vi "LXY_step.vi"() -> ()   [LabVIEW 2019]
uses:
  lib/Keithley 622x/Configure/2182 -A/Low Level/Typedefs/KE2182 -- Voltage Ranges.ctl
  lib/Keithley 622x/Configure/2182 -A/Low Level/Typedefs/KE2182 -- Filter Type.ctl
  lib/Keithley 622x/Configure/2182 -A/Low Level/Typedefs/KE2182 -- Filter Count.ctl
  lib/Keithley 622x/Configure/2182 -A/Low Level/Typedefs/KE2182 -- Filter Window.ctl
  lib/Keithley 622x/Configure/2182 -A/Low Level/Typedefs/KE2182 -- NPLCs.ctl
  lib/Keithley 622x/Configure/Delta PDelta DCon Modes/Typedefs/KE622x -- Delta Mode Params.ctl
  lib/Keithley 622x/Configure/Delta PDelta DCon Modes/Low Level/Typedefs/KE622x -- Delta PDelta Mode High Level.ctl
  lib/Keithley 622x/Configure/Delta PDelta DCon Modes/Low Level/Typedefs/KE622x -- Delta PDelta Mode Low Level.ctl
  lib/Keithley 622x/Configure/Delta PDelta DCon Modes/Low Level/Typedefs/KE622x -- Delta DCon Mode Delay.ctl
  lib/Keithley 622x/Configure/Delta PDelta DCon Modes/Low Level/Typedefs/KE622x -- Delta PDelta Mode Num Cycles Mode.ctl
  lib/Keithley 622x/Configure/Delta PDelta DCon Modes/Low Level/Typedefs/KE622x -- Delta PDelta Mode Num Cycles.ctl
  SubVI/ctl/config.ctl
  <vilib>/NI/Modbus Library/API/Master/Modbus Master.lvclass
  SubVI/ctl/initialize.ctl
  SubVI/ctl/Instrument.ctl
  SubVI/ctl/Instrument Type.ctl
  D:/measure/lib/QDInstrument.dll
  lib/QDInstrument.dll
  SubVI/ctl/335 state.ctl
  SubVI/ctl/limit.ctl
  SubVI/ctl/9T mag field stauts.ctl
  SubVI/ctl/warning.ctl
  lib/Keithley 622x/Keithley 622x.lvlib
panel:
  in  "config":T1={"initialize"=enum."SR830", "6221"={"6221 Resource"="GPIB0::24::INSTR", "Delta status"=FALSE, "电流|RMS(A)"=0.0}, "SR830+6221"={"source"=0, "Current(A)"=0.0, "阻抗(Ohm)"=0.0, "SR830 1"=FALSE, "SR830 2"=FALSE, "SR830 3"=FALSE, "SR830 4"=FALSE, "VISA 1"="", "VISA 2"="", "VISA 3"="", "VISA 4"="", "Reserve 1"=0, "Reserve 2"=-1, "Reserve 3"=-1, "Reserve 4"=-1, "Sensitivity 1"=-1, "Sensitivity 2"=0, "Sensitivity 3"=-1, "Sensitivity 4"=-1, "量程入 1"=0, "量程入 2"=0, "量程入 3"=0, "量程入 4"=0}, "2400"={"2400"=FALSE, "VISA"=""}, "ch"={"ch"=[], "current"=[], "change?"=[], "holding current\nwhen change ch?"=FALSE}, "Instrument"={"335 Resource"="GPIB0::24::INSTR", "Input (0:A)"=0, "Instrument Type"=enum."SVSM", "quantum design"=refnum, "Heater Output (1:1)"=1, "semaphore"=refnum, "TCP master instance"=refnum, "335 Status"=refnum, "M24C Resource"="GPIB0::24::INSTR", "4G supply"="GPIB0::24::INSTR", "Temp Status 24C"=refnum, "Temp"=refnum, "9T信号"=refnum, "limit"={"Field limit"=0.0, "Field rate limit"=0.0, "Temp limit"=0.0, "Temp low limit"=0.0, "Temp rate limit "=0.0}, "4g supply status"=refnum, "vi路径"=""}, "Aborting"=refnum, "数据文件"=refnum, "warning"=refnum, "2614B"={"2614B chA"=FALSE, "2614B chB"=FALSE, "VISA"=""}, "33522b"={"33522b resource name"=""}} {"Instrument"."Input (0:A)" items=["A", "B"]; "Instrument"."Heater Output (1:1)" items=["1"=1, "2"=2]; "SR830+6221"."Sensitivity 4" items=["Auto Gain"=-1, "2 nV/fA"=0, "5 nV/fA"=1, "10 nV/fA"=2, "20 nV/fA"=3, "50 nV/fA"=4, "100 nV/fA"=5, "200 nV/fA"=6, "500 nV/fA"=7, "1 uV/pA"=8, "2 uV/pA"=9, "5 uV/pA"=10, "10 uV/pA"=11, "20 uV/pA"=12, "50 uV/pA"=13, "100 uV/pA"=14, "200 uV/pA"=15, "500 uV/pA"=16, "1 mV/nA"=17, "2 mV/nA"=18, "5 mV/nA"=19, "10 mV/nA"=20, "20 mV/nA"=21, "50 mV/nA"=22, "100 mV/nA"=23, "200 mV/nA"=24, "500 mV/mA"=25, "1 V/uA"=26]; "SR830+6221"."Sensitivity 3" items=["Auto Gain"=-1, "2 nV/fA"=0, "5 nV/fA"=1, "10 nV/fA"=2, "20 nV/fA"=3, "50 nV/fA"=4, "100 nV/fA"=5, "200 nV/fA"=6, "500 nV/fA"=7, "1 uV/pA"=8, "2 uV/pA"=9, "5 uV/pA"=10, "10 uV/pA"=11, "20 uV/pA"=12, "50 uV/pA"=13, "100 uV/pA"=14, "200 uV/pA"=15, "500 uV/pA"=16, "1 mV/nA"=17, "2 mV/nA"=18, "5 mV/nA"=19, "10 mV/nA"=20, "20 mV/nA"=21, "50 mV/nA"=22, "100 mV/nA"=23, "200 mV/nA"=24, "500 mV/mA"=25, "1 V/uA"=26]; "SR830+6221"."Sensitivity 1" items=["Auto Gain"=-1, "2 nV/fA"=0, "5 nV/fA"=1, "10 nV/fA"=2, "20 nV/fA"=3, "50 nV/fA"=4, "100 nV/fA"=5, "200 nV/fA"=6, "500 nV/fA"=7, "1 uV/pA"=8, "2 uV/pA"=9, "5 uV/pA"=10, "10 uV/pA"=11, "20 uV/pA"=12, "50 uV/pA"=13, "100 uV/pA"=14, "200 uV/pA"=15, "500 uV/pA"=16, "1 mV/nA"=17, "2 mV/nA"=18, "5 mV/nA"=19, "10 mV/nA"=20, "20 mV/nA"=21, "50 mV/nA"=22, "100 mV/nA"=23, "200 mV/nA"=24, "500 mV/mA"=25, "1 V/uA"=26]; "SR830+6221"."Sensitivity 2" items=["Auto Gain"=-1, "2 nV/fA"=0, "5 nV/fA"=1, "10 nV/fA"=2, "20 nV/fA"=3, "50 nV/fA"=4, "100 nV/fA"=5, "200 nV/fA"=6, "500 nV/fA"=7, "1 uV/pA"=8, "2 uV/pA"=9, "5 uV/pA"=10, "10 uV/pA"=11, "20 uV/pA"=12, "50 uV/pA"=13, "100 uV/pA"=14, "200 uV/pA"=15, "500 uV/pA"=16, "1 mV/nA"=17, "2 mV/nA"=18, "5 mV/nA"=19, "10 mV/nA"=20, "20 mV/nA"=21, "50 mV/nA"=22, "100 mV/nA"=23, "200 mV/nA"=24, "500 mV/mA"=25, "1 V/uA"=26]; "SR830+6221"."Reserve 4" items=["Auto Gain"=-1, "2 nV/fA"=0, "5 nV/fA"=1, "10 nV/fA"=2, "20 nV/fA"=3, "50 nV/fA"=4, "100 nV/fA"=5, "200 nV/fA"=6, "500 nV/fA"=7, "1 uV/pA"=8, "2 uV/pA"=9, "5 uV/pA"=10, "10 uV/pA"=11, "20 uV/pA"=12, "50 uV/pA"=13, "100 uV/pA"=14, "200 uV/pA"=15, "500 uV/pA"=16, "1 mV/nA"=17, "2 mV/nA"=18, "5 mV/nA"=19, "10 mV/nA"=20, "20 mV/nA"=21, "50 mV/nA"=22, "100 mV/nA"=23, "200 mV/nA"=24, "500 mV/mA"=25, "1 V/uA"=26]; "SR830+6221"."Reserve 3" items=["Auto Reserve"=-1, "High Reserve"=0, "Normal"=1, "Low Noise"=2]; "SR830+6221"."Reserve 2" items=["Auto Reserve"=-1, "High Reserve"=0, "Normal"=1, "Low Noise"=2]; "SR830+6221"."Reserve 1" items=["Auto Reserve"=-1, "High Reserve"=0, "Normal"=1, "Low Noise"=2]; "SR830+6221"."source" items=["SR830 1", "SR830 2", "SR830 3", "SR830 4"]}
  in  "间隔":dbl=4.0
  in  "最小电压":dbl=-48.0
  in  "最大电压":dbl=148.0
  in  "零电压":dbl
  in  "2400 配置电流":dbl=1e-05
  out "电压数组":dbl[](array[numeric])
  in  "Delta Mode Params In":T7={"High Level (A)"=0.001, "Low Level (A)"=-0.001, "Delay (s)"=0.002, "Num Cycles Mode"=enum."Finite Count", "Finite Count"=10, "Abort On\nCompliance?"=FALSE, "Cold Swithing\nMode Enabled?"=FALSE} {"Finite Count" min=1 max=65536; "Low Level (A)" min=-0.105 max=0.0 format="%.3p"; "High Level (A)" min=0.0 max=0.105 format="%.3p"; "Delay (s)" min=0.001 max=9999.999 format="%.3f"}
  in  "2812 -A Params In":T18={"Auto Range?"=FALSE, "Man / Selected\nRange"=enum."10mV", "Enable Digital\nFilter?"=FALSE, "Filter Type"=enum."Moving", "Filter Count"=10, "Filter\nWindow (%)"=0.01, "Enable Analog\nFilter?"=FALSE, "NPLCs"=5} {"Filter\nWindow (%)" min=0.0 max=10.0 step=0.01 format="%.2f"; "Filter Count" min=1 max=100; "NPLCs" min=1 max=10}
  in  "2400 Compliance  Level":dbl=0.0001 format="%#_13g"
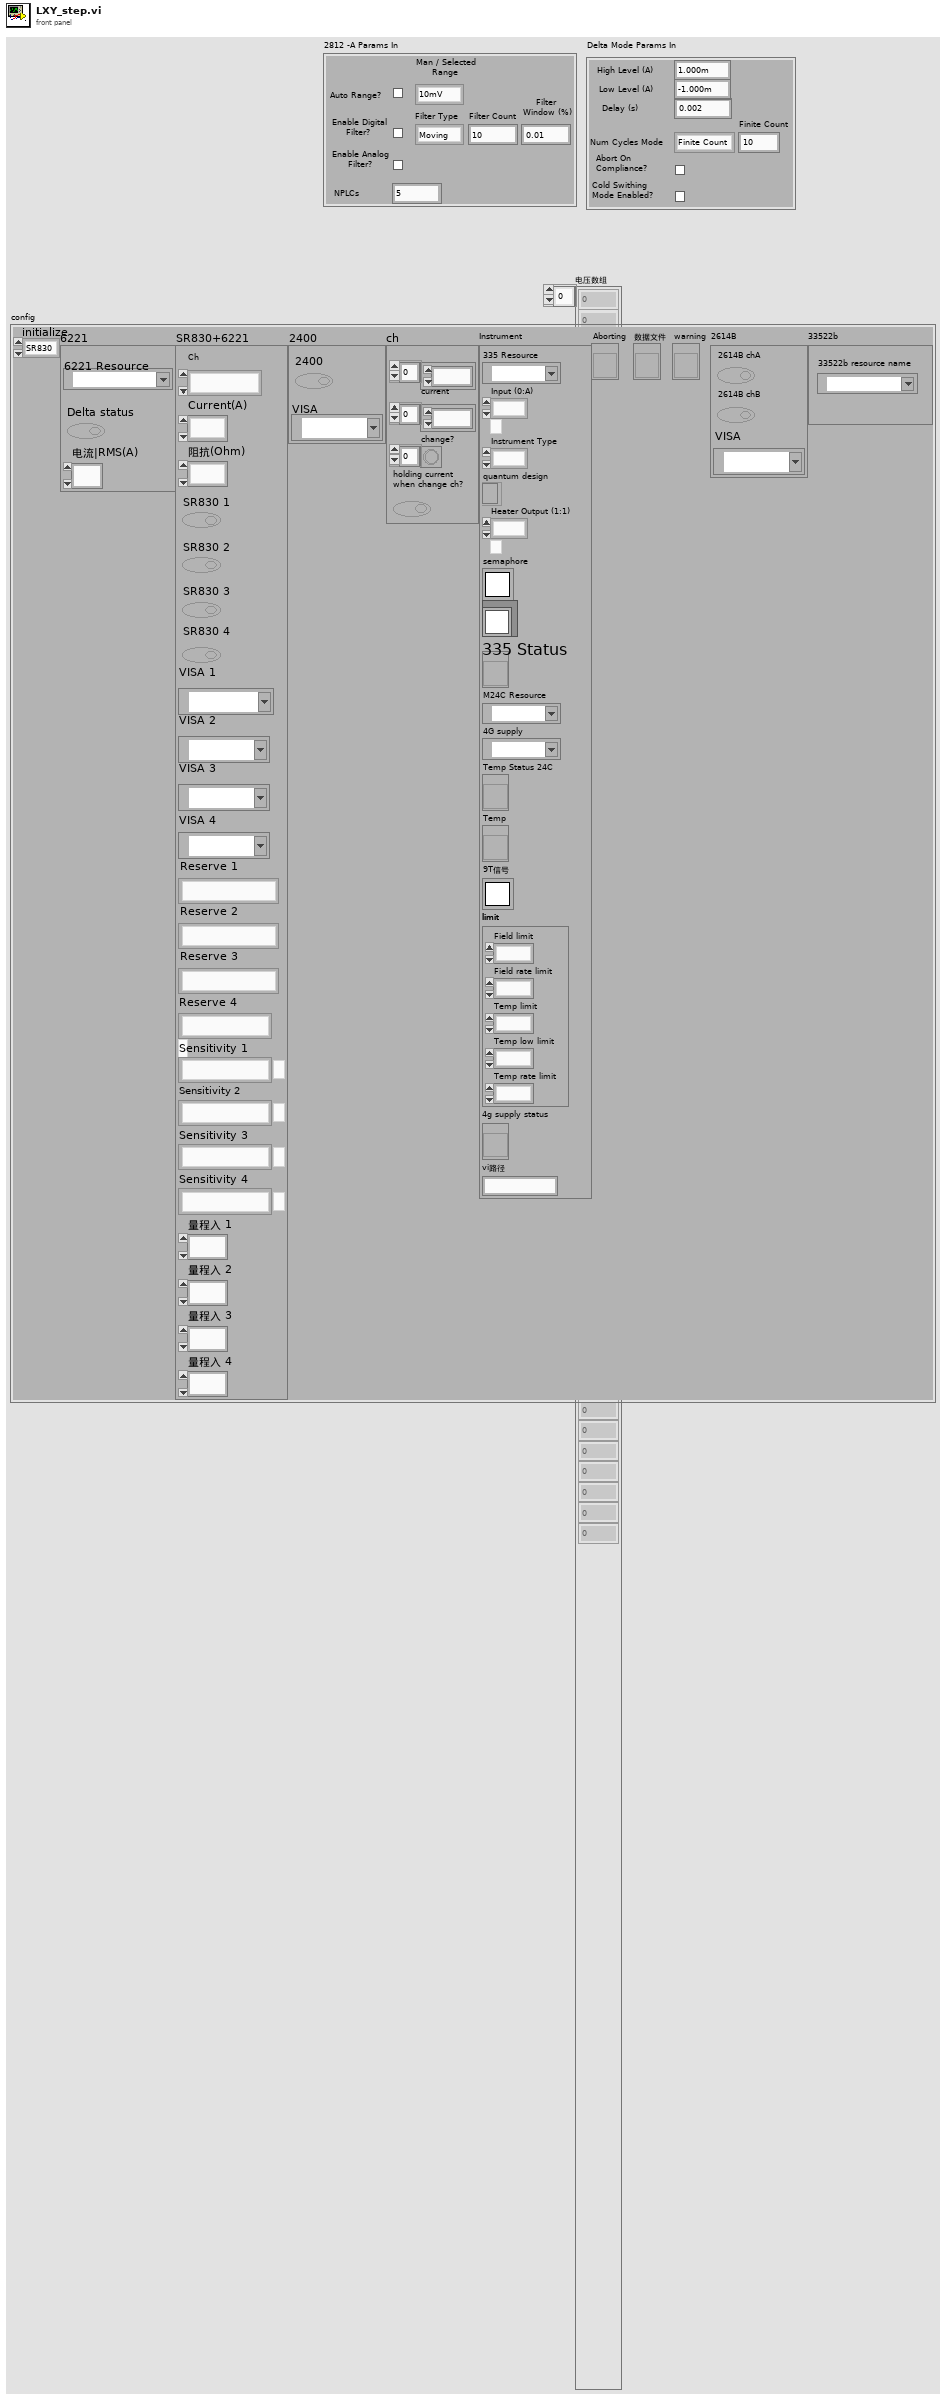
[diagram p1: front panel]
types:
  T1 = typedef "config.ctl" = cluster{"initialize":T2, "6221":cluster{"6221 Resource":refnum<visa-resource-name>, "Delta status":bool, "电流|RMS(A)":dbl}, "SR830+6221":cluster{"source":u16, "Current(A)":dbl, "阻抗(Ohm)":dbl, "SR830 1":bool, "SR830 2":bool, "SR830 3":bool, "SR830 4":bool, "VISA 1":refnum<visa-resource-name>, "VISA 2":refnum<visa-resource-name>, "VISA 3":refnum<visa-resource-name>, "VISA 4":refnum<visa-resource-name>, "Reserve 1":i16, "Reserve 2":i16, "Reserve 3":i16, "Reserve 4":i16, "Sensitivity 1":i16, "Sensitivity 2":i16, "Sensitivity 3":i16, "Sensitivity 4":i16, "量程入 1":i32, "量程入 2":i32, "量程入 3":i32, "量程入 4":i32}, "2400":cluster{"2400":bool, "VISA":refnum<visa-resource-name>}, "ch":cluster{"ch":i32[], "current":dbl[], "change?":bool[], "holding current\nwhen change ch?":bool}, "Instrument":T3, "Aborting":refnum<vi>, "数据文件":refnum<vi>, "warning":refnum<vi>, "2614B":cluster{"2614B chA":bool, "2614B chB":bool, "VISA":refnum<visa-resource-name>}, "33522b":cluster{"33522b resource name":refnum<visa-resource-name>}}
  T2 = typedef "initialize.ctl" = enum16{"SR830", "keithley6221-SR830", "Delta", "Delta-tunnelling", "keithley6221-2182-DC", "33522b"}
  T3 = typedef "Instrument.ctl" = cluster{"335 Resource":refnum<visa-resource-name>, "Input (0:A)":u16, "Instrument Type":T4, "quantum design":refnum<k24>, "Heater Output (1:1)":u16, "semaphore":T5, "TCP master instance":refnum<class "Modbus Master.lvclass">, "335 Status":refnum<vi>, "M24C Resource":refnum<visa-resource-name>, "4G supply":refnum<visa-resource-name>, "Temp Status 24C":refnum<vi>, "Temp":refnum<vi>, "9T信号":T5, "limit":T6, "4g supply status":refnum<vi>, "vi路径":string}
  T4 = typedef "Instrument Type.ctl" = enum16{"PPMS", "VersaLab", "DynaCool", "SVSM", "PPMS-Rotate", "Lakeshore335", "9T mag"}
  T5 = typedef "Semaphore RefNum" = refnum<k1>
  T6 = typedef "limit.ctl" = cluster{"Field limit":dbl, "Field rate limit":dbl, "Temp limit":dbl, "Temp low limit":dbl, "Temp rate limit ":dbl}
  T7 = typedef "Keithley 622x.lvlib/KE622x -- Delta Mode Params.ctl" = cluster{"High Level (A)":T8, "Low Level (A)":T9, "Delay (s)":T10, "Num Cycles Mode":T11, "Finite Count":T12, "Abort On\nCompliance?":bool, "Cold Swithing\nMode Enabled?":bool}
  T8 = typedef "Keithley 622x.lvlib/KE622x -- Delta PDelta Mode High Level.ctl" = dbl
  T9 = typedef "Keithley 622x.lvlib/KE622x -- Delta PDelta Mode Low Level.ctl" = dbl
  T10 = typedef "Keithley 622x.lvlib/KE622x -- Delta DCon Mode Delay.ctl" = dbl
  T11 = typedef "Keithley 622x.lvlib/KE622x -- Delta PDelta Mode Num Cycles Mode.ctl" = enum16{"Finite Count", "Infinite"}
  T12 = typedef "Keithley 622x.lvlib/KE622x -- Delta PDelta Mode Num Cycles.ctl" = u32
  T13 = typedef "Keithley 622x.lvlib/KE2182 -- Voltage Ranges.ctl" = enum16{"10mV", "100mV", "1V", "10V", "100V"}
  T14 = typedef "Keithley 622x.lvlib/KE2182 -- Filter Type.ctl" = enum16{"Moving", "Repeat"}
  T15 = typedef "Keithley 622x.lvlib/KE2182 -- Filter Count.ctl" = u32
  T16 = typedef "Keithley 622x.lvlib/KE2182 -- Filter Window.ctl" = dbl
  T17 = typedef "Keithley 622x.lvlib/KE2182 -- NPLCs.ctl" = u32
  T18 = cluster{"Auto Range?":bool, "Man / Selected\nRange":T13, "Enable Digital\nFilter?":bool, "Filter Type":T14, "Filter Count":T15, "Filter\nWindow (%)":T16, "Enable Analog\nFilter?":bool, "NPLCs":T17}
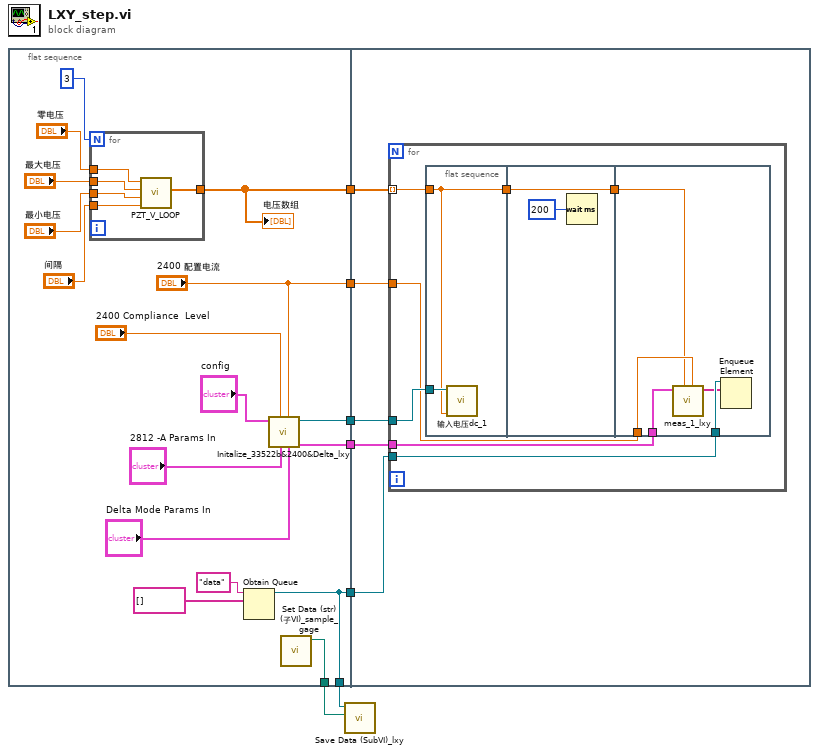
[diagram p0: block diagram]
diagram:
  n1 = flat-sequence {
    tunnel: [w19] -> w7
    tunnel: [w19] -> w6
    tunnel: [w18] -> w5
    tunnel: [w17] -> w4
    tunnel: [w15] -> w3
    tunnel: ["2400 配置电流"] -> w2
    tunnel: [w8] -> w1
    tunnel: w7 -> [w33]
    tunnel: w4 -> [w34]
    tunnel: w3 -> [w32]
    tunnel: w2 -> [w31]
    tunnel: w1 -> [w30]
    frame #0 {
      n2 = for {
        N: 3 -> [_]
        tunnel: [w29] -> w15
        tunnel: "零电压" -> [w28]
        tunnel: "最大电压" -> [w27]
        tunnel: "最小电压" -> [w26]
        tunnel: "间隔" -> [w25]
        n3 = call "PZT_V_LOOP.vi"("间隔"=w25, "最小电压"=w26, "最大电压"=w27, "零电压"=w28) -> ("output array"=w29:dbl[])  [unwired: 7 in]
      }
      "电压数组" <- w15
      n4 = Obtain Queue(name (unnamed)="data", element data type=string[] [] ("数组")) -> (queue out=w19:refnum<queue>)  [unwired: 3 in, 2 out]
      n5 = call "Initalize_33522b&2400&Delta_lxy.vi"("Delta Mode Params In"="Delta Mode Params In", "Output Level (0)"="2400 配置电流", "2812 -A Params In"="2812 -A Params In", "Compliance  Level (0.1)"="2400 Compliance  Level", "config"="config") -> ("输出簇"=w8:T1, "33522b resource name 2"=w17:refnum<visa-resource-name>)  [unwired: 5 in]
      n6 = call "Set Data (str) (子VI)_sample_gage.vi"() -> ("path"=w18:path)  [unwired: 10 in, 1 out]
    }
    frame #1 {
      n7 = for {
        tunnel: w34 -> [w41]
        tunnel: w33 -> [w40]
        tunnel: w32 -> [w39] mode=indexing
        tunnel: w31 -> [w38]
        tunnel: w30 -> [w35]
        n8 = flat-sequence {
          tunnel: w41 -> [w43]
          tunnel: w39 -> [w42]
          tunnel: [w42] -> w36
          tunnel: [w44] -> w37
          tunnel: w36 -> [w44]
          tunnel: w40 -> [w50]
          tunnel: w38 -> [w48]
          tunnel: w37 -> [w47]
          tunnel: w35 -> [w46]
          frame #0 {
            n9 = call "输入电压dc_1.vi"("压电陶瓷电压 (0.1 Vpp)"=w42, "33522b resource name"=w43) -> ()  [unwired: 5 in]
          }
          frame #1 {
            n10 = Wait (ms)(milliseconds to wait=u32 200 ("等待时间（毫秒）")) -> ()  [unwired: 1 out]
          }
          frame #2 {
            n11 = call "meas_1_lxy.vi"("Output Level (0)"=w48, "压电陶瓷电压 (0.1 Vpp)"=w47, "config"=w46) -> ("数组"=w49:string[])  [unwired: 6 in, 2 out]
            n12 = Enqueue Element(queue=w50, element=w49) -> ()  [unwired: 2 in, 3 out]
          }
        }
      }
    }
  }
  n13 = call "Save Data (SubVI)_lxy.vi"("path"=w5, "队列输入"=w6) -> ()  [unwired: 10 in]
